vi "Untitled 8 (SubVI).vi"(2 "error out 2":errorcluster, 3 "Protocol_Generic out 2":refnum<class "Protocol_Logging.lvclass">) -> (0 "error out":errorcluster, 1 "Protocol_Generic out":refnum<class "Protocol_Logging.lvclass">)   [LabVIEW 2010, in "Protocol_Logging.lvclass"]
uses:
  Protocol_Logging.lvclass
  Protocol_Logging.lvclass/Protocol_Logging.ctl
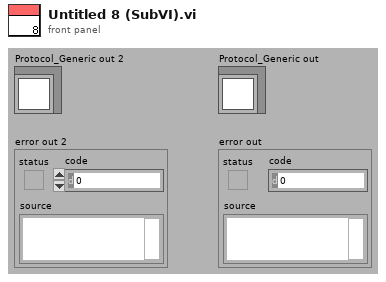
[diagram p1: front panel]
types:
  T1 = cluster{"Axis Information":cluster{"Device ID":i32, "Device Name":string, "Device Type":i32}[], "Axis Selector":i32[], "Control Modes out":u16[], "error out":errorcluster, "Channel Data":cluster{"Name":string, "Type":i32, "SI Full Scale":dbl, "Full Scale":dbl, "Units String":string, "Display Format":string, "Gauge Length":dbl}[][]}
  T2 = cluster{"Device ID":i32, "Device Name":string, "Device Type":i32}[]
  T3 = cluster{"Sample interval - ms (2)":dbl, "Buffer Length (1000)":i32, "No. of Buffers (0)":i32}
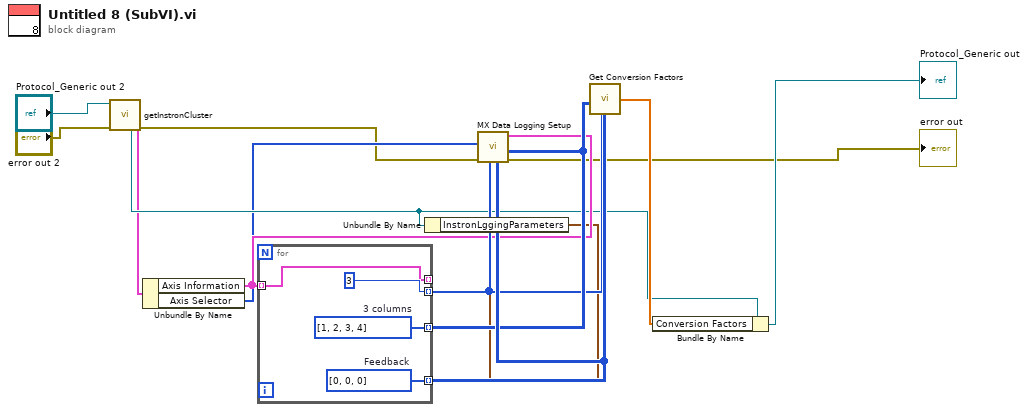
[diagram p0: block diagram]
diagram:
  n1 = call-dynamic "getInstronCluster.vi"("error in (no error)"="error out 2", "Protocol_Generic in"="Protocol_Generic out 2") -> ("error out"=w5:errorcluster, "InstronCluster"=w4:T1, "Protocol_Generic out"=w8:refnum<class "Protocol_Logging.lvclass">)  [unwired: 7 in]
  n2 = Unbundle By Name(w4) -> ("Axis Information"=w11:T2, "Axis Selector"=w7:i32[])
  n3 = for {
    tunnel: [w18] -> w13 mode=indexing
    tunnel: [w17] -> w14 mode=indexing
    tunnel: [3] -> w12 mode=indexing
    tunnel: [w15] -> _ mode=indexing
    tunnel: w11 -> [w15] mode=indexing
    w17 = i32[] [0, 0, 0]  # Feedback
    w18 = i32[] [1, 2, 3, 4]  # 3 columns
  }
  n4 = Unbundle By Name(w8) -> ("InstronLggingParameters"=w1:T3)
  n5 = call "MX Data Logging Setup.vi"("Column Types"=w14, "Number of Columns"=w12, "Interval/Buffer Parameters"=w1, "error in (no error)"=w5, "Column Channels"=w13, "Axis Selector"=w7, "Axis Information"=w11) -> ("error out"=→"error out":errorcluster)  [unwired: 3 out]
  n6 = call "Get Conversion Factors.vi"("Column Channels"=w13, "Column Types"=w14, "Number of Columns"=w12) -> ("Conversion Factors"=w10:dbl[])  [unwired: 2 in]
  n7 = Bundle By Name(cluster=w8, "Conversion Factors"=w10) -> (→"Protocol_Generic out":refnum<class "Protocol_Logging.lvclass">)
